vi "RT_Shut_Down_VI.vi"(8 "error in (no error)":errorcluster) -> ()   [LabVIEW 2020]
uses:
  <vilib>/dex/Flush And Wait Empty Condition.ctl
  <vilib>/FPGAPlugInAG/cRIO-9040/niLvFpga_Open_cRIO-9040.vi
  <vilib>/Utility/error.llb/Error Cluster From Error Code.vi
  <vilib>/rvi/errors/niLvFpgaAdjustHostInterfaceError.vi
  <vilib>/FPGAPlugInAG/cRIO-9040/niLvFpga_Close_cRIO-9040.vi
  <vilib>/rvi/interface/nirviOpenFPGA/nirviOpenFPGA.xnode
  FPGA Bitfiles/depapp_FPGATarget_FPGAmainsimplifi_tvdh8urvlFE.lvbitx
  FPGA_main_simplified.vi
  <vilib>/rvi/interface/nirviReadWriteControl/nirviReadWriteControl.xnode
  <vilib>/rvi/interface/nirviMethod/nirviMethod.xnode
  <vilib>/rvi/interface/nirviCloseFPGA/nirviCloseFPGA.xnode
  NiFpgaLv.dll
  <vilib>/FPGAPlugInAG/cRIO-9040/niLvFpga_StopFifo_cRIO-9040.vi
  <vilib>/rvi/errors/niLvFpgaMergeErrorWithErrorCode.vi
panel:
  in  "output cluster":T1
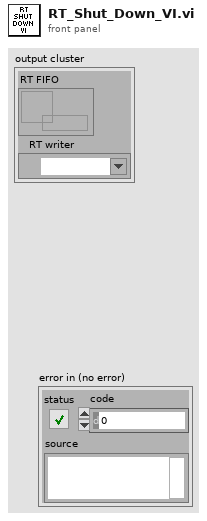
[diagram p1: front panel]
types:
  T1 = cluster{"RT FIFO":refnum<k33>, "RT writer":refnum<k21>}
  T2 = typedef "Flush And Wait Empty Condition.ctl" = u8
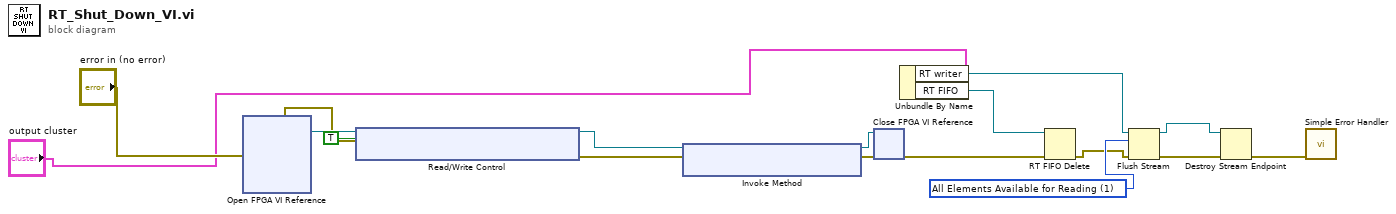
[diagram p0: block diagram]
diagram:
  w14 = T2 1 items=["All Elements Read From Stream", "All Elements Available for Reading"] ("wait condition")
  n1 = xnode "Open FPGA VI Reference"("error in"="error in (no error)") -> ("FPGA VI Reference Out"=w8:refnum<k20>, "error out"=w6:errorcluster)  [unwired: 1 in]
  n2 = xnode "Read/Write Control"("FPGA VI Reference In"=w8, "error in"=w6, "Stop"=TRUE) -> ("FPGA VI Reference Out"=w4:refnum<k20>, "error out"=w5:errorcluster)
  n3 = xnode "Invoke Method"("FPGA VI Reference In"=w4, "error in"=w5) -> ("FPGA VI Reference Out"=w12:refnum<k20>, "error out"=w13:errorcluster)
  n4 = xnode "Close FPGA VI Reference"("FPGA VI Reference In"=w12, "error in"=w13) -> ("error out"=w11:errorcluster)
  n5 = Unbundle By Name("output cluster") -> ("RT writer"=w17:refnum<k21>, "RT FIFO"=w9:refnum<k33>)
  n6 = RT FIFO Delete(0:w9, 3:w11) -> (11:w3:errorcluster)  [unwired: 1 in]
  n7 = Flush Stream(8:w3, 10:w14, 11:w17) -> (0:w2:errorcluster, 3:w15:refnum<k21>)  [unwired: 1 in, 1 out]
  n8 = Destroy Stream Endpoint(8:w2, 11:w15) -> (0:w1:errorcluster)
  n9 = call <vilib>:"Simple Error Handler.vi"("error in (no error)"=w1) -> ()  [unwired: 4 in, 5 out]
